vi "Convert Boolean to String.vi"(11 "Boolean":bool) -> (3 "String":string)   [LabVIEW 2020, in "MacroAssert.lvlib"]
doc: "Outputs a true/false string based on the input."
uses:
  MacroAssert.lvlib
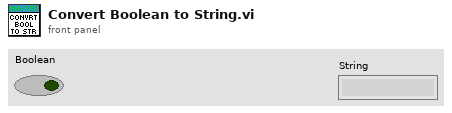
[diagram p1: front panel]
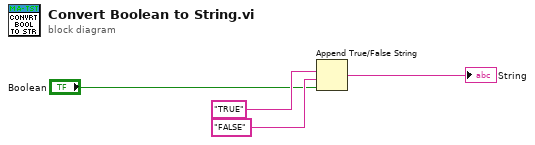
[diagram p0: block diagram]
diagram:
  n1 = Append True/False String(1:"Boolean", 2:"FALSE" ("false string"), 3:"TRUE" ("true string")) -> (0:→"String":string)  [unwired: 1 in]
